vi "WriteTxt2dv2.vi"() -> ()   [LabVIEW 2014]
uses:
  <vilib>/Utility/sysdir.llb/System Directory Type.ctl
panel:
  in  "Filename":string
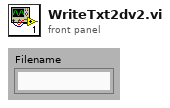
[diagram p1: front panel]
types:
  T1 = typedef "System Directory Type.ctl" = i32
  T2 = enum16{"open", "replace", "create", "open or create", "replace or create", "replace or create with confirmation"}
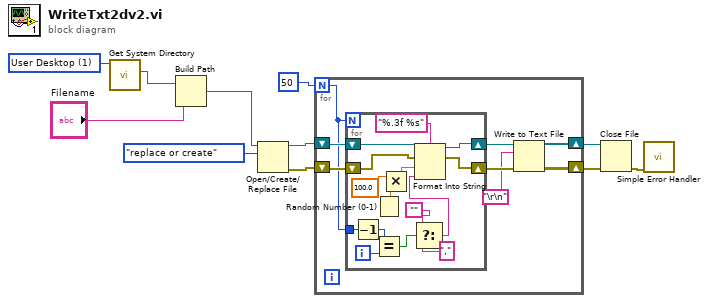
[diagram p0: block diagram]
diagram:
  w4 = T1 1 items=["User Home"=0, "User Desktop"=1, "User Documents"=2, "User Application Data"=3, "User Preferences"=4, "User Temporary"=5, "Public Documents"=6, "Public Application Data"=7, "Public Preferences"=8, "Public Cache"=13, "System Core Libraries"=9, "System Installed Libraries"=10, "Application Files"=11, "Boot Volume Root"=12] ("system directory type")
  n1 = call <vilib>:"Get System Directory.vi"("system directory type"=w4) -> ("system directory"=w3:path)  [unwired: 10 in]
  n2 = Build Path(base path=w3, name or relative path="Filename") -> (appended path=w1:path)
  n3 = Open/Create/Replace File(file path (use dialog)=w1, operation (0:open)=T2."replace or create") -> (refnum out=w10:refnum<file>, error out=w9:errorcluster)  [unwired: 4 in, 1 out]
  n4 = for {
    N: 50 -> [w17]
    shift-right: [w13] -> w7
    shift-left: w10 -> [w19]
    shift-right: [w15] -> w8
    shift-left: w9 -> [w18]
    n5 = for {
      N: w17 -> [_]
      shift-right: [w32] -> w16
      shift-left: w18 -> [w31]
      shift-right: [w33] -> w14
      shift-left: w19 -> [w34]
      tunnel: w17 -> [w26]
      i -> [w25]
      n6 = Decrement(x=w26) -> (x-1=w24:i32)
      n7 = Random Number (0-1)() -> (number: 0 to 1=w30:dbl)
      n8 = Equal?(x=w24, y=w25) -> (x = y?=w23:bool)
      n9 = Multiply(x=100.0, y=w30) -> (x*y=w28:dbl)
      n10 = Select(t="", s=w23, f=",") -> (s? t:f=w21:string)
      n11 = Format Into String(format string="%.3f %s", initial string=w34, error in=w31, w28, w21) -> (resulting string=w33:refnum<file>, error out=w32:errorcluster)
    }
    n12 = Write to Text File(file (use dialog)=w14, text="\r\n", error in=w16) -> (refnum out=w13:refnum<file>, error out=w15:errorcluster)  [unwired: 1 in, 1 out]
  }
  n13 = Close File(refnum=w7, error in=w8) -> (error out=w6:errorcluster)  [unwired: 1 out]
  n14 = call <vilib>:"Simple Error Handler.vi"("error in (no error)"=w6) -> ()  [unwired: 4 in, 5 out]
